vi "setTiming.vi"(2 "error in (no error)":errorcluster, 3 "SoundAO in":refnum<class "SoundAO.lvclass">) -> (0 "error out":errorcluster, 1 "SoundAO out":refnum<class "SoundAO.lvclass">)   [LabVIEW 2011, in "Hardware.lvlib" / "Channels.lvlib" / "SoundAO.lvclass"]
doc: "Abstract Methods.\n\nUse this vi to set the timing and triggering information for the analog output channel."
uses:
  SoundAO.lvclass
  AnalogOutput.lvclass
  <vilib>/sound2/lvsound2.llb/Sound Output Set Volume (Single).vi
  <vilib>/sound2/lvsound2.llb/Sampling Mode.ctl
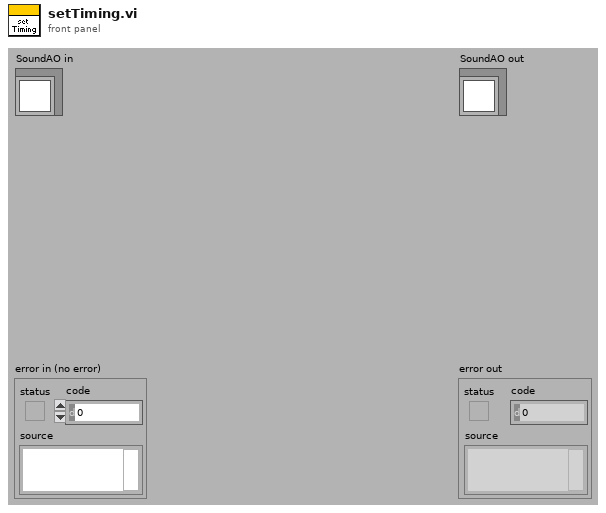
[diagram p1: front panel]
types:
  T1 = cluster{"Clock source":string, "Clock rate":dbl, "Start trigger line":string, "Sample Rate":dbl, "Sample No.":dbl}
  T2 = typedef "Sampling Mode.ctl" = i32
  T3 = typedef "Sound Output Task ID.ctl" = u32
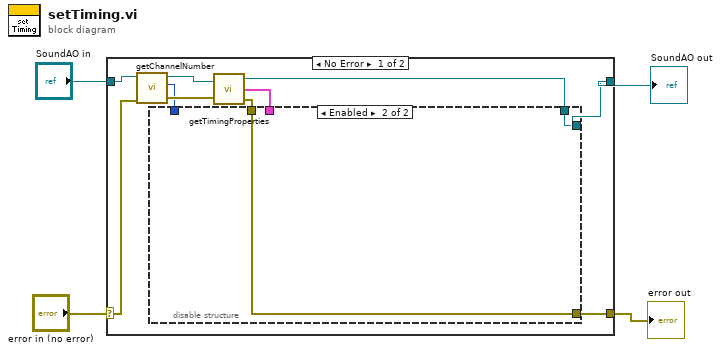
[diagram p0: block diagram]
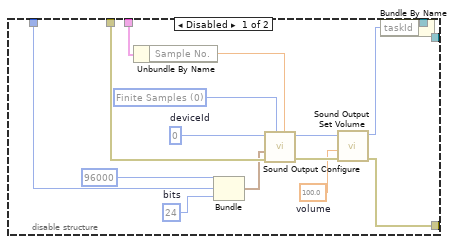
[diagram p2: hidden frame]
diagram:
  n1 = case shown="No Error" "error in (no error)" {
    selector: "error in (no error)" -> [w9 w33]
    tunnel: [w7 w33] -> w3
    tunnel: "SoundAO in" -> [w10 w34]
    tunnel: [w5 w34] -> w1
    frame No Error {
      n2 = call "getChannelNumber.vi"("error in (no error)"=w9, "SoundAO in"=w10) -> ("error out"=w11:errorcluster, "numberOfChannels"=w8:i32, "SoundAO out"=w12:refnum<class "SoundAO.lvclass">)  [unwired: 7 in]
      n3 = call "getTimingProperties.vi"("AnalogOutput.lvclass in"=w12, "error in (no error)"=w11) -> ("AnalogOutput.lvclass out"=w6:refnum<class "SoundAO.lvclass">, "Timing"=w14:T1, "error out"=w13:errorcluster)
      n4 = disable-structure shown="Enabled" {
        disable-tunnel: w14 -> [w30 _]
        disable-tunnel: w13 -> [w26 w32]
        disable-tunnel: w8 -> [w22 _]
        disable-tunnel: [w19 w32] -> w7
        disable-tunnel: w6 -> [w17 w31]
        disable-tunnel: [w15 w31] -> w5
        frame Disabled {
          w20 = 100.0  # volume
          w21 = 24  # bits
          w25 = T2 0 items=["Finite Samples", "Continuous Samples"] ("sample mode")
          w29 = 0  # deviceId
          n5 = Unbundle By Name(w30) -> ("Sample No."=w24:dbl)
          n6 = Bundle(96000, "numberOfChannels"=w22, "bits"=w21) -> (w23:cluster{i32, "numberOfChannels":i32, "bits":i32})  [unwired: 1 in]
          n7 = call <vilib>:"Sound Output Configure.vi"("number of samples/ch"=w24, "sample mode"=w25, "error in (no error)"=w26, "sound format"=w23, "device ID"=w29) -> ("error out"=w27:errorcluster, "task ID"=w28:T3)  [unwired: 5 in]
          n8 = call-poly <vilib>:"Sound Output Set Volume.vi"("error in (no error)"=w27, "volume"=w20, "task ID"=w28) -> ("error out"=w19:errorcluster, "task ID out"=w16:T3)  [unwired: 7 in]
          n9 = Bundle By Name(cluster=w17, "taskId"=w16) -> (w15:refnum<class "SoundAO.lvclass">)
        }
        frame Enabled {
        }
      }
    }
    frame Error {
    }
  }
  "error out" <- w3
  "SoundAO out" <- w1
